vi "DEMO.vi"() -> ()   [LabVIEW 2018]
uses:
  MELSEC Communication Protocol/Data Def/Mitsubishi_Batch Read In Word Units Command.ctl
  MELSEC Communication Protocol/Data Def/Mitsubishi_Device Code.ctl
  MELSEC Communication Protocol/Data Def/Mitsubishi_Registers Data Type.ctl
  MELSEC Communication Protocol/Data Def/Mitsubishi_Request Message Format.ctl
  MELSEC Communication Protocol/Data Def/Mitsubishi_Access Route.ctl
  MELSEC Communication Protocol/Data Def/Mitsubishi_Request Type.ctl
panel:
  in  "Polling Time(ms)":i32=10 min=10
  in  "Port":u16=2000
  in  "IP Adress":string="192.168.1.250"
  in  "Recording File Path":path=path "C:/DEMO.csv"
  in  "Stop":bool
  in  "Record":bool
  in  "Connect":bool
  in  "Batch Read In Word Units":T1={"Head Device Number"=0, "Device Code"=168, "Number Of Device Point"=1, "Registers Data Type"=enum."16 Bit int"} {"Device Code" items=["SM"=145, "SD"=169, "X*"=156, "Y*"=157, "M*"=144, "L*"=146, "F*"=147, "V*"=148, "B*"=160, "D*"=168, "W*"=180, "TS"=193, "TC"=192, "TN"=194, "SS"=199, "SC"=198, "SN"=200, "CS"=196, "CC"=195, "CN"=197, "SB"=161, "SW"=181, "S*"=152, "DX"=162, "DY"=163, "Z*"=204, "R*"=175, "ZR"=176, "G"=171]; "Number Of Device Point" min=1 max=10}
  out "Waveform Chart":T4(graph)
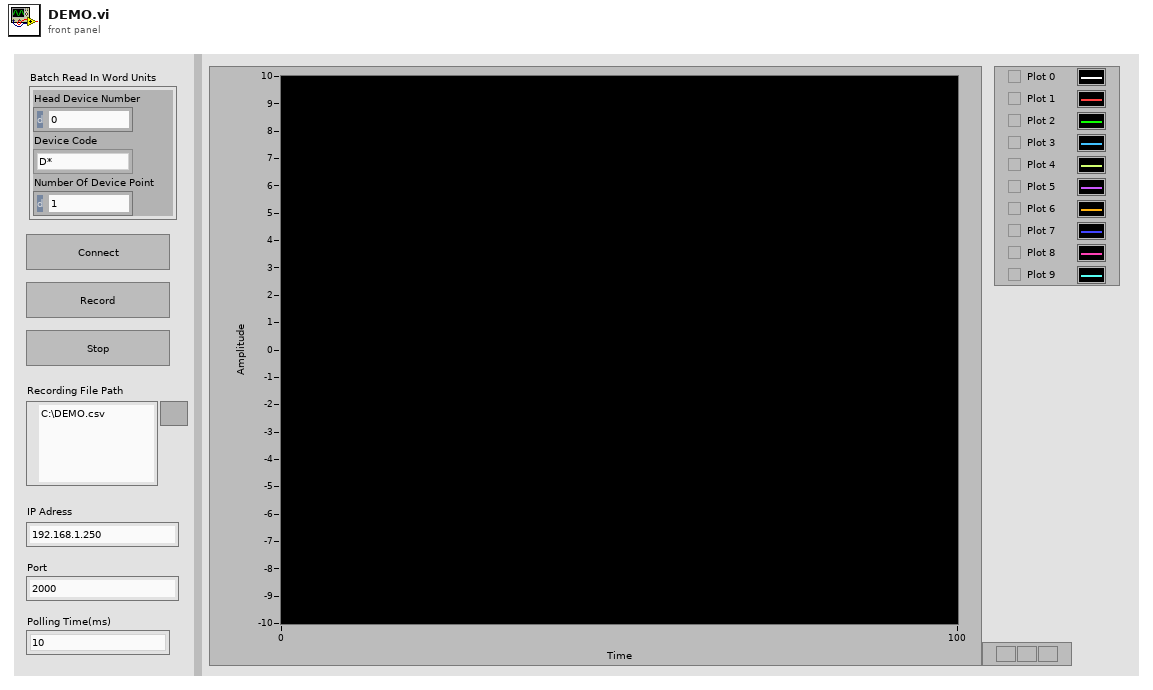
[diagram p1: front panel]
types:
  T1 = typedef "Mitsubishi_Batch Read In Word Units Command.ctl" = cluster{"Head Device Number":u16, "Device Code":T2, "Number Of Device Point":u16, "Registers Data Type":T3}
  T2 = typedef "Mitsubishi_Device Code.ctl" = u8
  T3 = typedef "Mitsubishi_Registers Data Type.ctl" = enum16{"16 Bit int", "16 Bit Uint", "32 Bit int", "32 Bit Uint", "32 Bit float", "64 Bit double", "Characters"}
  T4 = cluster{"Response Data[0]":i16, "Response Data[1]":i16, "Response Data[2]":i16, "Response Data[3]":i16, "Response Data[4]":i16, "Response Data[5]":i16, "Response Data[6]":i16, "Response Data[7]":i16, "Response Data[8]":i16, "Response Data[9]":i16}
  T5 = enum16{"Standard", "Buffered", "CRLF", "Immediate"}
  T6 = typedef "Mitsubishi_Request Message Format.ctl" = cluster{"Access Route":T7, "Monitoring Timer(ms)":u16, "Request Type":T8, "Request Data":variant}
  T7 = typedef "Mitsubishi_Access Route.ctl" = cluster{"Network No.":string, "PC No.":string, "Module I/O No.":string, "Module Station No.":string}
  T8 = typedef "Mitsubishi_Request Type.ctl" = enum16{"Batch read in word units", "Batch write in word units"}
  T9 = enum16{"open", "replace", "create", "open or create", "replace or create", "replace or create with confirmation"}
  T10 = typedef "Mitsubishi_Read Response Message.ctl" = cluster{"Subheader":u16, "Access Route":cluster{"Network No.":u8, "PC No.":u8, "Module I/O No.":u16, "Module Station No.":u8}, "Response Data Length":u8, "End Code":u16, "Response Data":i16[]}
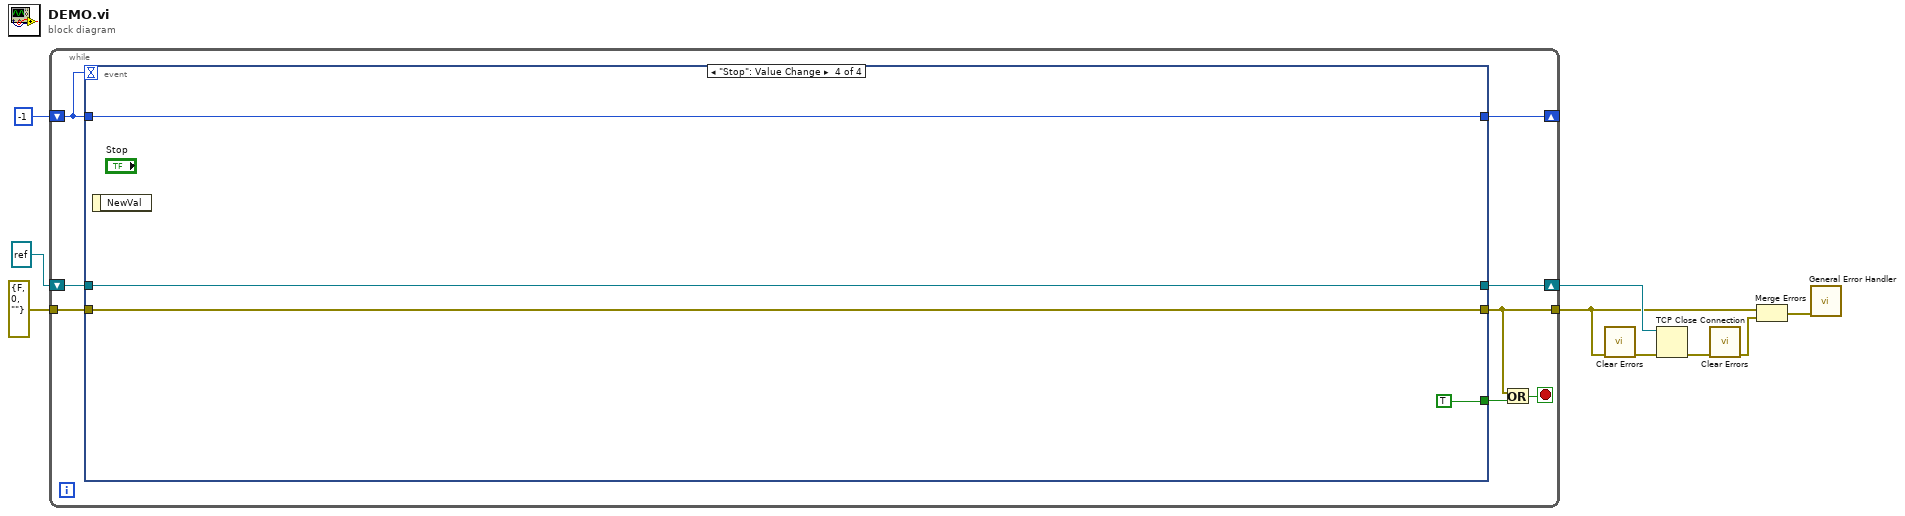
[diagram p0: block diagram]
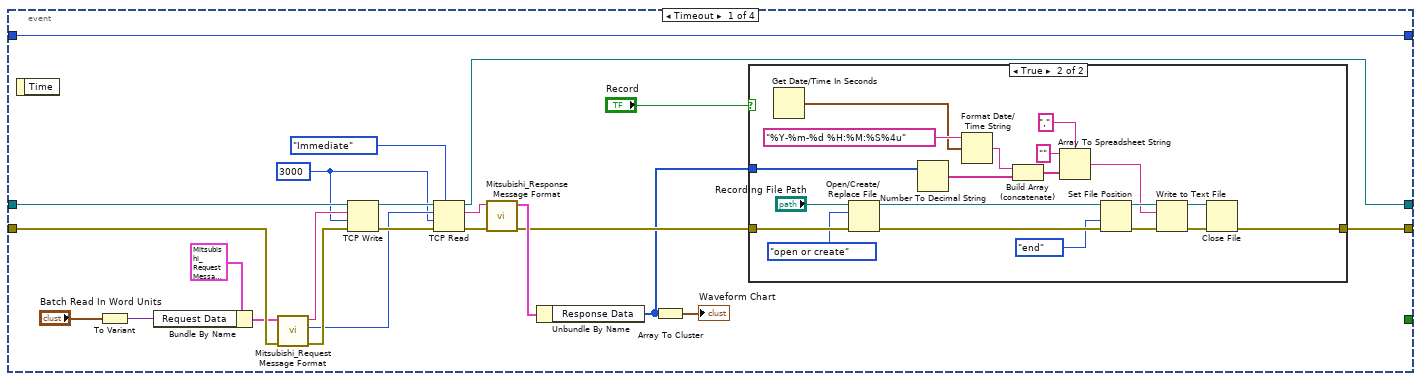
[diagram p2: hidden frame]
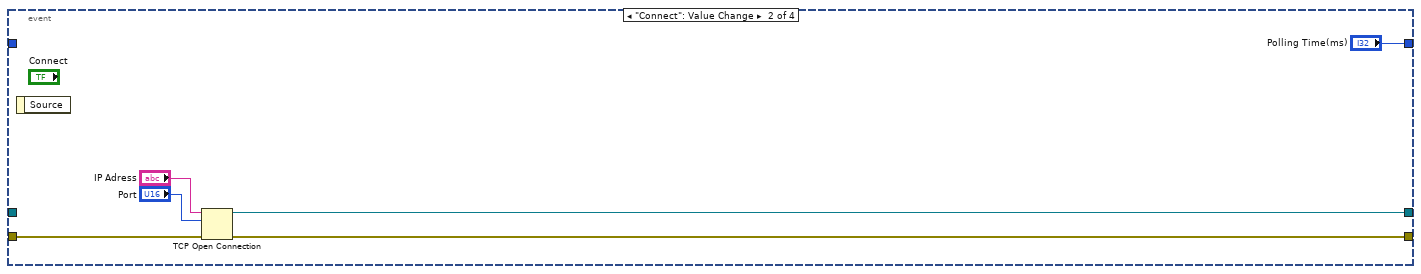
[diagram p4: hidden frame]
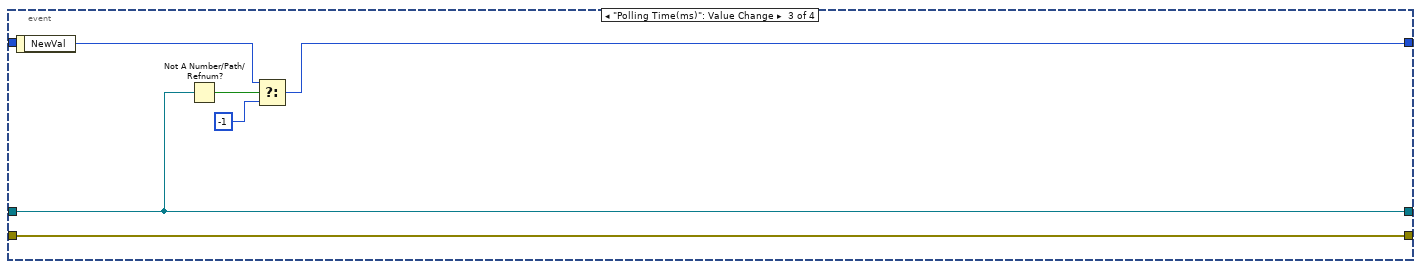
[diagram p5: hidden frame]
diagram:
  n1 = while {
    tunnel: errorcluster {"status"=FALSE, "code"=0, "source"=""} ("error constant") -> [w17]
    tunnel: [w11] -> w4
    shift-right: [w16] -> w5
    shift-left: refnum<k5> refnum ("connection ID") -> [w13]
    shift-right: [w14] -> _
    shift-left: -1 -> [w15]
    stop <- w10 stop-if-true
    n2 = event shown="[3] \"Stop\": Value Change" {
      selector: _ -> [_ _ _ _]
      dyn-events: _ -> [_ _ _ _]
      timeout: w15 -> [_ _ _ _]
      tunnel: [w19 w66 w73 w76] -> w11
      tunnel: w17 -> [w39 w65 w73 w76]
      tunnel: [w18 w64 w72 w75] -> w16
      tunnel: w15 -> [w40 _ _ w77]
      tunnel: [w40 "Polling Time(ms)" w68 w77] -> w14
      tunnel: w13 -> [w34 _ w72 w75]
      tunnel: [_ _ _ TRUE] -> w12
      event Timeout {
        w28 = 3000 ("timeout ms (25000)")
        n3 = event-data() -> ()  [unwired: 1 in, 1 out]
        n4 = To Variant(anything="Batch Read In Word Units") -> (Variant=w36:variant)
        n5 = Bundle By Name(cluster=T6 {"Access Route"={"Network No."="\u0000", "PC No."="ÿ", "Module I/O No."="\u0003", "Module Station No."="\u0000"}, "Monitoring Timer(ms)"=4000, "Request Type"=enum."Batch read in word units", "Request Data"=variant} ("Message Format"), "Request Data"=w36) -> (w35:T6)
        n6 = call "Mitsubishi_Request Message Format.vi"("error in"=w39, "Request Message Format"=w35) -> ("error out"=w32:errorcluster, "Byte To Read"=w29:i32, "Request Message"=w33:string)  [unwired: 7 in]
        n7 = TCP Write(connection ID=w34, data in=w33, error in (no error)=w32, 9:w28) -> (connection ID out=w30:refnum<k5>, error out=w31:errorcluster)  [unwired: 1 out]
        n8 = TCP Read(connection ID=w30, bytes to read=w29, error in (no error)=w31, 7:T5."Immediate" ("mode (standard)"), 9:w28) -> (connection ID out=w18:refnum<k5>, data out=w25:string, error out=w26:errorcluster)
        n9 = call "Mitsubishi_Response Message Format.vi"("error in"=w26, "Respond Data"=w25) -> ("error out"=w22:errorcluster, "Response Message"=w24:T10)  [unwired: 8 in]
        n10 = Unbundle By Name(w24) -> ("Response Data"=w20:i16[])
        n11 = Array To Cluster(array=w20) -> (cluster=→"Waveform Chart":T4)
        n12 = case shown="True" "Record" {
          tunnel: w22 -> [w41 w61]
          tunnel: w20 -> [_ w56]
          tunnel: [w41 w42] -> w19
          frame False {
          }
          frame True {
            n13 = Get Date/Time In Seconds() -> (seconds since 1Jan1904=w57:timestamp)
            n14 = Open/Create/Replace File(file path (use dialog)="Recording File Path", error in=w61, operation (0:open)=T9."open or create") -> (refnum out=w50:refnum<file>, error out=w49:errorcluster)  [unwired: 3 in, 1 out]
            n15 = Number To Decimal String(number=w56) -> (decimal integer string=w54:string[])  [unwired: 1 in]
            n16 = Format Date/Time String(time format string (%c)="%Y-%m-%d %H:%M:%S%4u", seconds (now)=w57) -> (date/time string=w55:string)  [unwired: 1 in]
            n17 = Build Array (concatenate)(w55, w54) -> (w53:string[])
            n18 = Array To Spreadsheet String(delimiter (Tab)=",", array=w53, 3:"" ("format string")) -> (spreadsheet string=w45:string)
            n19 = Set File Position(refnum=w50, from (0:start)=enum16{"start", "end", "current"}."end", error in=w49) -> (refnum out=w46:refnum<file>, error out=w47:errorcluster)  [unwired: 1 in]
            n20 = Write to Text File(file (use dialog)=w46, text=w45, error in=w47) -> (refnum out=w43:refnum<file>, error out=w44:errorcluster)  [unwired: 1 in, 1 out]
            n21 = Close File(refnum=w43, error in=w44) -> (error out=w42:errorcluster)  [unwired: 1 out]
          }
        }
      }
      event "Connect": Value Change {
        n22 = event-data() -> ()  [unwired: 1 in, 1 out]
        n23 = TCP Open Connection(address="IP Adress", remote port or service name="Port", error in (no error)=w65) -> (connection ID=w64:refnum<k5>, error out=w66:errorcluster)  [unwired: 2 in]
      }
      event "Polling Time(ms)": Value Change {
        n24 = event-data() -> ("NewVal"=w70:i32)  [unwired: 1 in]
        n25 = Not A Number/Path/Refnum?(number/path/refnum=w72) -> (NaN/Path/Refnum?=w71:bool)
        n26 = Select(t=w70, s=w71, f=-1) -> (s? t:f=w68:i32)
      }
      event "Stop": Value Change {
        n27 = event-data() -> ()  [unwired: 1 in, 1 out]
      }
    }
    n28 = Or(x=w11, y=w12) -> (x .or. y?=w10:bool)
  }
  n29 = call <vilib>:"Clear Errors.vi"("error in (no error)"=w4) -> ("error out"=w6:errorcluster)  [unwired: 5 in, 1 out]
  n30 = TCP Close Connection(connection ID=w5, error in (no error)=w6) -> (error out=w3:errorcluster)  [unwired: 1 in, 1 out]
  n31 = call <vilib>:"Clear Errors.vi"("error in (no error)"=w3) -> ("error out"=w2:errorcluster)  [unwired: 5 in, 1 out]
  n32 = Merge Errors(w4, w2) -> (w1:errorcluster)
  n33 = call <vilib>:"General Error Handler.vi"("error in (no error)"=w1) -> ()  [unwired: 10 in, 5 out]
